vi "_ClassManager_LoadClass.vi"(8 "error in (no error)":errorcluster, 10 "ClassPath":path) -> (0 "error out":errorcluster, 3 "Library Refnum out":refnum<vi>)   [LabVIEW 2014, in "_ClassManager.lvlib" / "_ClassManager.lvclass"]
uses:
  _ClassManager.lvclass
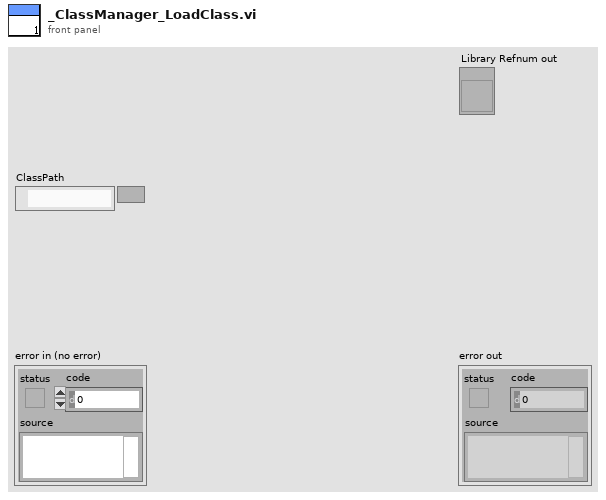
[diagram p1: front panel]
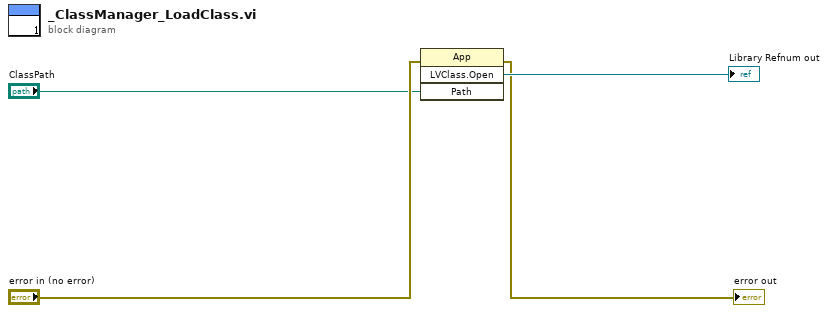
[diagram p0: block diagram]
diagram:
  n1 = invoke class="App" method="LVClass.Open"(error in="error in (no error)", "Path"="ClassPath") -> (error out=→"error out":errorcluster, "LVClass.Open"=→"Library Refnum out":refnum<vi>)  [unwired: 2 in, 2 out]
